vi "poll sockets.vi"(8 "error in":errorcluster, 10 "timeout":i32, 11 "sockets in":T1[](array[typedef])) -> (0 "error out":errorcluster, 3 "sockets out":T1[](array[typedef]))   [LabVIEW 2013, in "lvnano.lvlib"]
doc: "NN_EXPORT int nn_poll (struct nn_pollfd *fds, int nfds, int timeout);"
uses:
  lvnano.lvlib
  poll settings.ctl
  get last error code.vi
  get error string from code.vi
  <vilib>/Utility/error.llb/Error Cluster From Error Code.vi
  lvnanomsg.dll
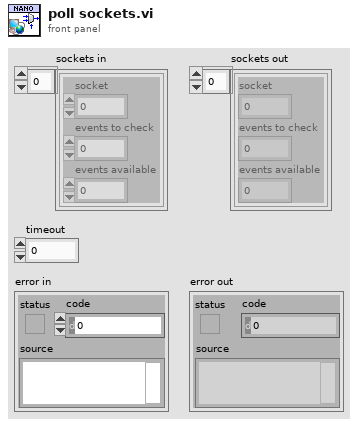
[diagram p1: front panel]
types:
  T1 = typedef "lvnano.lvlib/poll settings.ctl" = cluster{"socket":i32, "events to check":u16, "events available":u16}
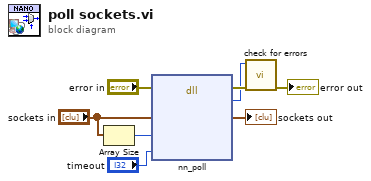
[diagram p0: block diagram]
diagram:
  n1 = Array Size(array="sockets in") -> (size(s)=w3:i32)
  n2 = dll-call lib="C:/Users/Daniel/Documents/nanomsg/lvnano/lvnanomsg.*" fn="nn_poll"(error in="error in", "sockets"="sockets in", "count"=w3, "timeout"="timeout") -> (error out=w6:errorcluster, "event count"=w4:i32, "sockets"=→"sockets out":T1[])  [unwired: 4 in, 1 out]
  n3 = call "check for errors.vi"("error in"=w6, "function return"=w4) -> ("error out"=→"error out":errorcluster)  [unwired: 9 in]
